vi "Write Data.vi"(8 "error in (no error)":errorcluster, 9 "Publication Time":timestamp, 10 "Value":variant, 11 "StreamToDiskTransport In":refnum<class "StreamToDiskTransport.lvclass">) -> (0 "error out":errorcluster, 3 "StreamToDiskTransport Out":refnum<class "StreamToDiskTransport.lvclass">)   [LabVIEW 2017, in "StreamToDiskTransport.lvclass"]
doc: "<License>\nCopyright © 2017 Composed Systems, LLC | All rights reserved\nwww.composed.io\n\nAuthor: Ethan Stern <ethan.stern@composed.io>\n\nThis software is provided \"AS IS\" WITHOUT WARRANTIES, either express or implied, AND IS FOR EDUCATIONAL PURPOSES ONLY.\n</License>"
uses:
  StreamToDiskTransport.lvclass
  StreamToDiskTransport.lvclass/StreamToDiskTransport.ctl
  <vilib>/Utility/error.llb/Error Cluster From Error Code.vi
  <vilib>/ErrorRing/Error Ring.xnode
  <vilib>/Utility/Data Type/NI_Data Type.lvlib
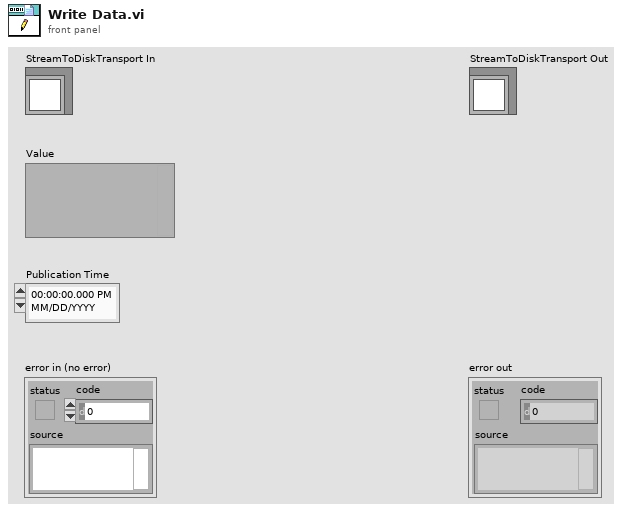
[diagram p1: front panel]
types:
  T1 = typedef "NI_Data Type.lvlib/Data Type.ctl" = enum8{"Invalid Type", "Void", "I8", "I16", "I32", "I64", "U8", "U16", "U32", "U64", "Single Float", "Double Float", "Extended Float", "Single Complex", "Double Complex", "Extended Complex", "Enum U8", "Enum U16", "Enum U32", "Enum U64", "Single Float With Unit", "Double Float With Unit", "Extended Float With Unit", "Single Complex with Unit", "Double Complex with Unit", "Extended Complex with Unit", "Boolean", "String", "Path", "Picture", "Tag", "Array", "Cluster", "Variant", "LV Variant", "Waveform", "Timestamp", "Digital Waveform", "Digital Data", "ExpressData", "Refnum", "External Data", "VI", "Poly VI", "LabVIEW Class Instance", "Fixed Point"}
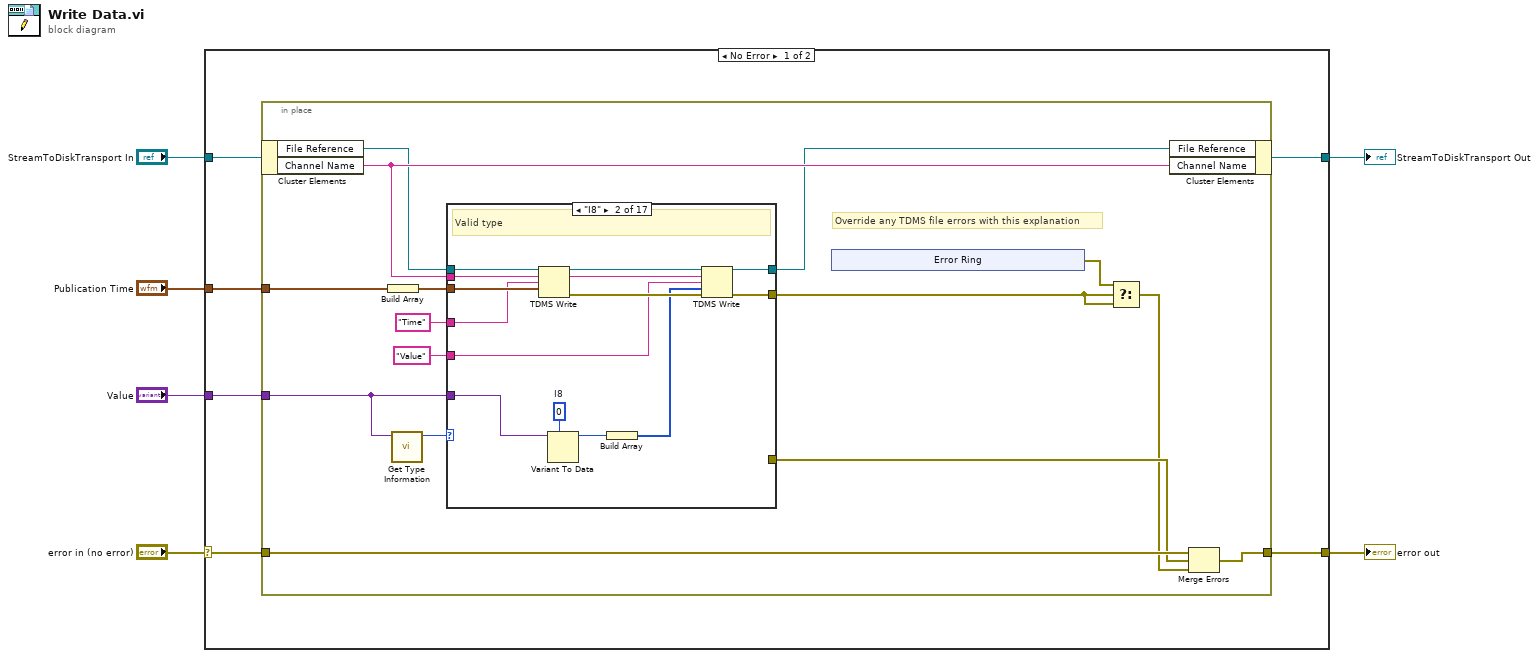
[diagram p0: block diagram]
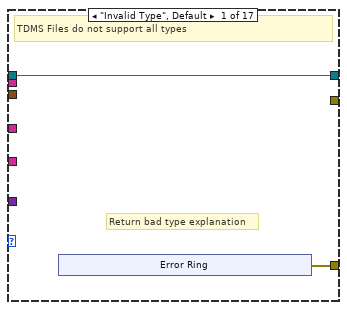
[diagram p2: hidden frame]
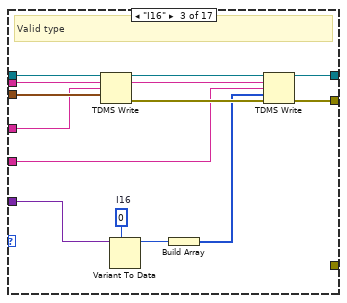
[diagram p3: hidden frame]
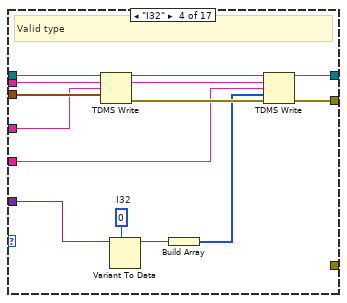
[diagram p4: hidden frame]
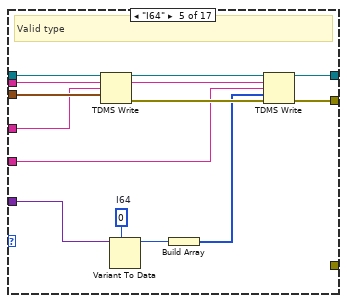
[diagram p5: hidden frame]
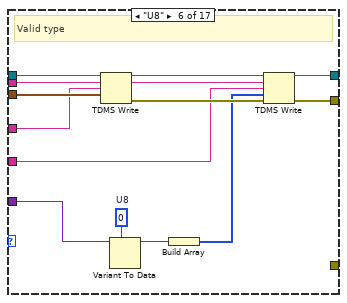
[diagram p6: hidden frame]
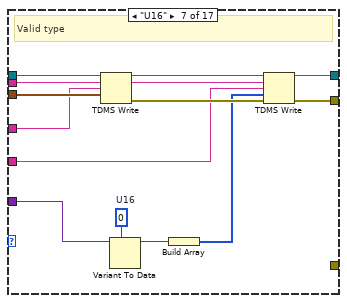
[diagram p7: hidden frame]
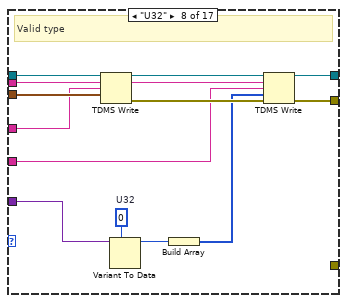
[diagram p8: hidden frame]
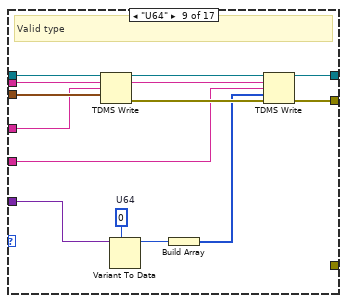
[diagram p9: hidden frame]
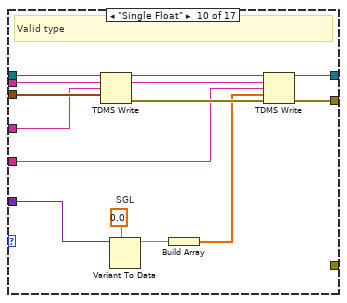
[diagram p10: hidden frame]
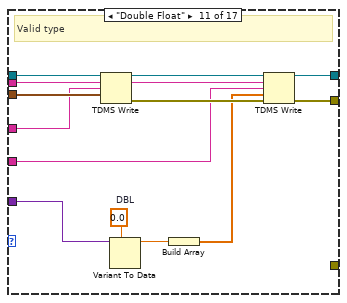
[diagram p11: hidden frame]
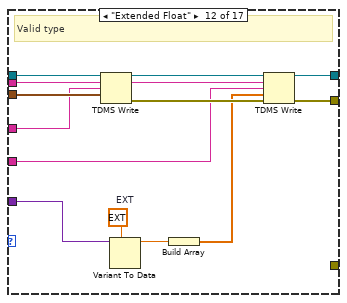
[diagram p12: hidden frame]
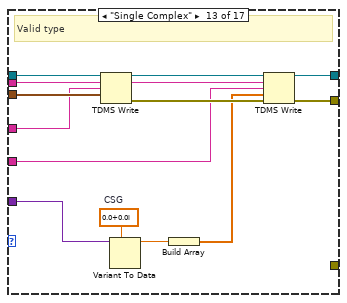
[diagram p13: hidden frame]
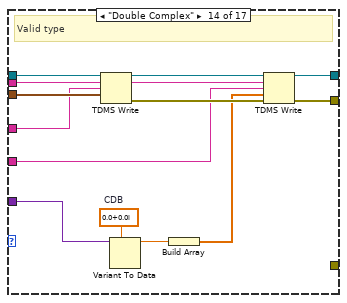
[diagram p14: hidden frame]
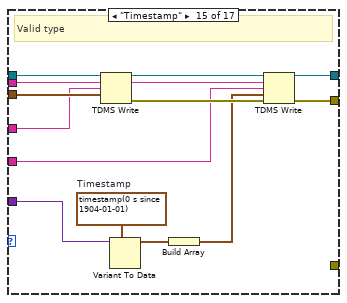
[diagram p15: hidden frame]
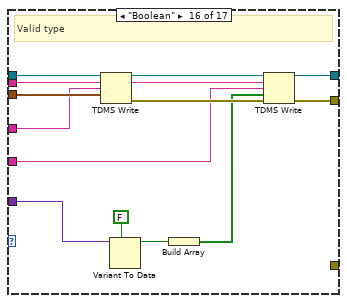
[diagram p16: hidden frame]
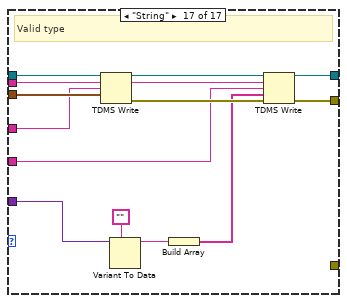
[diagram p17: hidden frame]
diagram:
  n1 = case shown="No Error" "error in (no error)" {
    selector: "error in (no error)" -> [w9 w264]
    tunnel: [w12 w264] -> w6
    tunnel: "Publication Time" -> [w11 _]
    tunnel: "Value" -> [w10 _]
    tunnel: "StreamToDiskTransport In" -> [w8 w265]
    tunnel: [w7 w265] -> w1
    frame No Error {
      n2 = in-place {
        in-place-border: [w26] -> w12
        in-place-border: w11 -> [w25]
        in-place-border: w10 -> [w24]
        in-place-border: w9 -> [w27]
        # "Override any TDMS file errors with this explanation"
        n3 = in-place-cluster #1(w8) -> ("File Reference"=w13:refnum<k34>, "Channel Name"=w21:string)
        n4 = Build Array(w25) -> (w19:timestamp[])
        n5 = call <vilib>:"Get Type Information.vi"("Variant"=w24) -> ("Type"=w23:T1)  [unwired: 6 in, 4 out]
        n6 = case shown="\"I8\"" w23 {
          tunnel: [_ w52 w66 w80 w94 w108 w122 w136 w150 w164 w178 w192 w206 w220 w234 w248 w262] -> w17
          tunnel: w21 -> [_ w43 w57 w71 w85 w99 w113 w127 w141 w155 w169 w183 w197 w211 w225 w239 w253]
          tunnel: w24 -> [_ w48 w62 w76 w90 w104 w118 w132 w146 w160 w174 w188 w202 w216 w230 w244 w258]
          tunnel: w13 -> [w34 w45 w59 w73 w87 w101 w115 w129 w143 w157 w171 w185 w199 w213 w227 w241 w255]
          tunnel: "Value" ("channel name(s) in (Untitled)") -> [_ w49 w63 w77 w91 w105 w119 w133 w147 w161 w175 w189 w203 w217 w231 w245 w259]
          tunnel: [w34 w46 w60 w74 w88 w102 w116 w130 w144 w158 w172 w186 w200 w214 w228 w242 w256] -> w14
          tunnel: "Time" ("channel name(s) in (Untitled)") -> [_ w40 w54 w68 w82 w96 w110 w124 w138 w152 w166 w180 w194 w208 w222 w236 w250]
          tunnel: w19 -> [_ w41 w55 w69 w83 w97 w111 w125 w139 w153 w167 w181 w195 w209 w223 w237 w251]
          tunnel: [w33 _ _ _ _ _ _ _ _ _ _ _ _ _ _ _ _] -> w18
          frame "Invalid Type", Default {
            # "Return bad type explanation"
            # "TDMS Files do not support all types"
            n7 = xnode "Error Ring"() -> ("error out"=w33:errorcluster)
          }
          frame "I8" {
            w50 = i8 0  # I8
            # "Valid type"
            n8 = TDMS Write(0:w45, 5:w43, 7:w40, 9:w41) -> (4:w44:refnum<k34>, 6:w42:string, 15:w53:errorcluster)  [unwired: 2 in, 1 out]
            n9 = Variant To Data(type=w50, Variant=w48) -> (data=w47:i8)  [unwired: 1 in, 1 out]
            n10 = Build Array(w47) -> (w51:i8[])
            n11 = TDMS Write(0:w44, 5:w42, 7:w49, 9:w51, 11:w53) -> (4:w46:refnum<k34>, 15:w52:errorcluster)  [unwired: 1 in, 2 out]
          }
          frame "I16" {
            w64 = i16 0  # I16
            # "Valid type"
            n12 = TDMS Write(0:w59, 5:w57, 7:w54, 9:w55) -> (4:w58:refnum<k34>, 6:w56:string, 15:w67:errorcluster)  [unwired: 2 in, 1 out]
            n13 = Variant To Data(type=w64, Variant=w62) -> (data=w61:i16)  [unwired: 1 in, 1 out]
            n14 = Build Array(w61) -> (w65:i16[])
            n15 = TDMS Write(0:w58, 5:w56, 7:w63, 9:w65, 11:w67) -> (4:w60:refnum<k34>, 15:w66:errorcluster)  [unwired: 1 in, 2 out]
          }
          frame "I32" {
            w78 = 0  # I32
            # "Valid type"
            n16 = TDMS Write(0:w73, 5:w71, 7:w68, 9:w69) -> (4:w72:refnum<k34>, 6:w70:string, 15:w81:errorcluster)  [unwired: 2 in, 1 out]
            n17 = Variant To Data(type=w78, Variant=w76) -> (data=w75:i32)  [unwired: 1 in, 1 out]
            n18 = Build Array(w75) -> (w79:i32[])
            n19 = TDMS Write(0:w72, 5:w70, 7:w77, 9:w79, 11:w81) -> (4:w74:refnum<k34>, 15:w80:errorcluster)  [unwired: 1 in, 2 out]
          }
          frame "I64" {
            w92 = i64 0  # I64
            # "Valid type"
            n20 = TDMS Write(0:w87, 5:w85, 7:w82, 9:w83) -> (4:w86:refnum<k34>, 6:w84:string, 15:w95:errorcluster)  [unwired: 2 in, 1 out]
            n21 = Variant To Data(type=w92, Variant=w90) -> (data=w89:i64)  [unwired: 1 in, 1 out]
            n22 = Build Array(w89) -> (w93:i64[])
            n23 = TDMS Write(0:w86, 5:w84, 7:w91, 9:w93, 11:w95) -> (4:w88:refnum<k34>, 15:w94:errorcluster)  [unwired: 1 in, 2 out]
          }
          frame "U8" {
            w106 = u8 0  # U8
            # "Valid type"
            n24 = TDMS Write(0:w101, 5:w99, 7:w96, 9:w97) -> (4:w100:refnum<k34>, 6:w98:string, 15:w109:errorcluster)  [unwired: 2 in, 1 out]
            n25 = Variant To Data(type=w106, Variant=w104) -> (data=w103:u8)  [unwired: 1 in, 1 out]
            n26 = Build Array(w103) -> (w107:u8[])
            n27 = TDMS Write(0:w100, 5:w98, 7:w105, 9:w107, 11:w109) -> (4:w102:refnum<k34>, 15:w108:errorcluster)  [unwired: 1 in, 2 out]
          }
          frame "U16" {
            w120 = u16 0  # U16
            # "Valid type"
            n28 = TDMS Write(0:w115, 5:w113, 7:w110, 9:w111) -> (4:w114:refnum<k34>, 6:w112:string, 15:w123:errorcluster)  [unwired: 2 in, 1 out]
            n29 = Variant To Data(type=w120, Variant=w118) -> (data=w117:u16)  [unwired: 1 in, 1 out]
            n30 = Build Array(w117) -> (w121:u16[])
            n31 = TDMS Write(0:w114, 5:w112, 7:w119, 9:w121, 11:w123) -> (4:w116:refnum<k34>, 15:w122:errorcluster)  [unwired: 1 in, 2 out]
          }
          frame "U32" {
            w134 = u32 0  # U32
            # "Valid type"
            n32 = TDMS Write(0:w129, 5:w127, 7:w124, 9:w125) -> (4:w128:refnum<k34>, 6:w126:string, 15:w137:errorcluster)  [unwired: 2 in, 1 out]
            n33 = Variant To Data(type=w134, Variant=w132) -> (data=w131:u32)  [unwired: 1 in, 1 out]
            n34 = Build Array(w131) -> (w135:u32[])
            n35 = TDMS Write(0:w128, 5:w126, 7:w133, 9:w135, 11:w137) -> (4:w130:refnum<k34>, 15:w136:errorcluster)  [unwired: 1 in, 2 out]
          }
          frame "U64" {
            w148 = u64 0  # U64
            # "Valid type"
            n36 = TDMS Write(0:w143, 5:w141, 7:w138, 9:w139) -> (4:w142:refnum<k34>, 6:w140:string, 15:w151:errorcluster)  [unwired: 2 in, 1 out]
            n37 = Variant To Data(type=w148, Variant=w146) -> (data=w145:u64)  [unwired: 1 in, 1 out]
            n38 = Build Array(w145) -> (w149:u64[])
            n39 = TDMS Write(0:w142, 5:w140, 7:w147, 9:w149, 11:w151) -> (4:w144:refnum<k34>, 15:w150:errorcluster)  [unwired: 1 in, 2 out]
          }
          frame "Single Float" {
            w162 = sgl 0.0  # SGL
            # "Valid type"
            n40 = TDMS Write(0:w157, 5:w155, 7:w152, 9:w153) -> (4:w156:refnum<k34>, 6:w154:string, 15:w165:errorcluster)  [unwired: 2 in, 1 out]
            n41 = Variant To Data(type=w162, Variant=w160) -> (data=w159:sgl)  [unwired: 1 in, 1 out]
            n42 = Build Array(w159) -> (w163:sgl[])
            n43 = TDMS Write(0:w156, 5:w154, 7:w161, 9:w163, 11:w165) -> (4:w158:refnum<k34>, 15:w164:errorcluster)  [unwired: 1 in, 2 out]
          }
          frame "Double Float" {
            w176 = 0.0  # DBL
            # "Valid type"
            n44 = TDMS Write(0:w171, 5:w169, 7:w166, 9:w167) -> (4:w170:refnum<k34>, 6:w168:string, 15:w179:errorcluster)  [unwired: 2 in, 1 out]
            n45 = Variant To Data(type=w176, Variant=w174) -> (data=w173:dbl)  [unwired: 1 in, 1 out]
            n46 = Build Array(w173) -> (w177:dbl[])
            n47 = TDMS Write(0:w170, 5:w168, 7:w175, 9:w177, 11:w179) -> (4:w172:refnum<k34>, 15:w178:errorcluster)  [unwired: 1 in, 2 out]
          }
          frame "Extended Float" {
            w190 = ext 0.0  # EXT
            # "Valid type"
            n48 = TDMS Write(0:w185, 5:w183, 7:w180, 9:w181) -> (4:w184:refnum<k34>, 6:w182:string, 15:w193:errorcluster)  [unwired: 2 in, 1 out]
            n49 = Variant To Data(type=w190, Variant=w188) -> (data=w187:ext)  [unwired: 1 in, 1 out]
            n50 = Build Array(w187) -> (w191:ext[])
            n51 = TDMS Write(0:w184, 5:w182, 7:w189, 9:w191, 11:w193) -> (4:w186:refnum<k34>, 15:w192:errorcluster)  [unwired: 1 in, 2 out]
          }
          frame "Single Complex" {
            w204 = csg 0.0+0.0i  # CSG
            # "Valid type"
            n52 = TDMS Write(0:w199, 5:w197, 7:w194, 9:w195) -> (4:w198:refnum<k34>, 6:w196:string, 15:w207:errorcluster)  [unwired: 2 in, 1 out]
            n53 = Variant To Data(type=w204, Variant=w202) -> (data=w201:csg)  [unwired: 1 in, 1 out]
            n54 = Build Array(w201) -> (w205:csg[])
            n55 = TDMS Write(0:w198, 5:w196, 7:w203, 9:w205, 11:w207) -> (4:w200:refnum<k34>, 15:w206:errorcluster)  [unwired: 1 in, 2 out]
          }
          frame "Double Complex" {
            w218 = cdb 0.0+0.0i  # CDB
            # "Valid type"
            n56 = TDMS Write(0:w213, 5:w211, 7:w208, 9:w209) -> (4:w212:refnum<k34>, 6:w210:string, 15:w221:errorcluster)  [unwired: 2 in, 1 out]
            n57 = Variant To Data(type=w218, Variant=w216) -> (data=w215:cdb)  [unwired: 1 in, 1 out]
            n58 = Build Array(w215) -> (w219:cdb[])
            n59 = TDMS Write(0:w212, 5:w210, 7:w217, 9:w219, 11:w221) -> (4:w214:refnum<k34>, 15:w220:errorcluster)  [unwired: 1 in, 2 out]
          }
          frame "Timestamp" {
            w232 = timestamp(0 s since 1904-01-01)  # Timestamp
            # "Valid type"
            n60 = TDMS Write(0:w227, 5:w225, 7:w222, 9:w223) -> (4:w226:refnum<k34>, 6:w224:string, 15:w235:errorcluster)  [unwired: 2 in, 1 out]
            n61 = Variant To Data(type=w232, Variant=w230) -> (data=w229:timestamp)  [unwired: 1 in, 1 out]
            n62 = Build Array(w229) -> (w233:timestamp[])
            n63 = TDMS Write(0:w226, 5:w224, 7:w231, 9:w233, 11:w235) -> (4:w228:refnum<k34>, 15:w234:errorcluster)  [unwired: 1 in, 2 out]
          }
          frame "Boolean" {
            # "Valid type"
            n64 = TDMS Write(0:w241, 5:w239, 7:w236, 9:w237) -> (4:w240:refnum<k34>, 6:w238:string, 15:w249:errorcluster)  [unwired: 2 in, 1 out]
            n65 = Variant To Data(type=FALSE, Variant=w244) -> (data=w243:bool)  [unwired: 1 in, 1 out]
            n66 = Build Array(w243) -> (w247:bool[])
            n67 = TDMS Write(0:w240, 5:w238, 7:w245, 9:w247, 11:w249) -> (4:w242:refnum<k34>, 15:w248:errorcluster)  [unwired: 1 in, 2 out]
          }
          frame "String" {
            # "Valid type"
            n68 = TDMS Write(0:w255, 5:w253, 7:w250, 9:w251) -> (4:w254:refnum<k34>, 6:w252:string, 15:w263:errorcluster)  [unwired: 2 in, 1 out]
            n69 = Variant To Data(type="", Variant=w258) -> (data=w257:string)  [unwired: 1 in, 1 out]
            n70 = Build Array(w257) -> (w261:string[])
            n71 = TDMS Write(0:w254, 5:w252, 7:w259, 9:w261, 11:w263) -> (4:w256:refnum<k34>, 15:w262:errorcluster)  [unwired: 1 in, 2 out]
          }
        }
        n72 = xnode "Error Ring"() -> ("error out"=w16:errorcluster)
        n73 = Select(t=w16, s=w17, f=w17) -> (s? t:f=w15:errorcluster)
        n74 = in-place-cluster #1("File Reference"=w14, "Channel Name"=w21) -> (w7:refnum<class "StreamToDiskTransport.lvclass">)
        n75 = Merge Errors(w27, w18, w15) -> (w26:errorcluster)
      }
    }
    frame Error {
    }
  }
  "error out" <- w6
  "StreamToDiskTransport Out" <- w1
